vi "RenderTexture.vi"(4 "dstrect":T1, 5 "Entire Rendering Target (F)":bool, 6 "srcrect":T1, 7 "Entire Texture (F)":bool, 8 "No Error":errorcluster, 10 "texture [SDL_Texture *]":i64, 11 "renderer [SDL_Renderer *]":i64) -> (0 "error out":errorcluster)   [LabVIEW 2024, in "SDL3.lvlib" / "Render.lvlib"]
doc: "<B>Summary</B>\nCopy a portion of the texture to the current rendering target at subpixel precision.\n\n<B>Thread Safety</B>\nYou may only call this function from the main thread."
uses:
  Render.lvlib
  Rect/FRect--cluster.ctl
  Error/Error.lvlib
  Lib/SDL3-32.dll
  Rect/Rect.lvlib
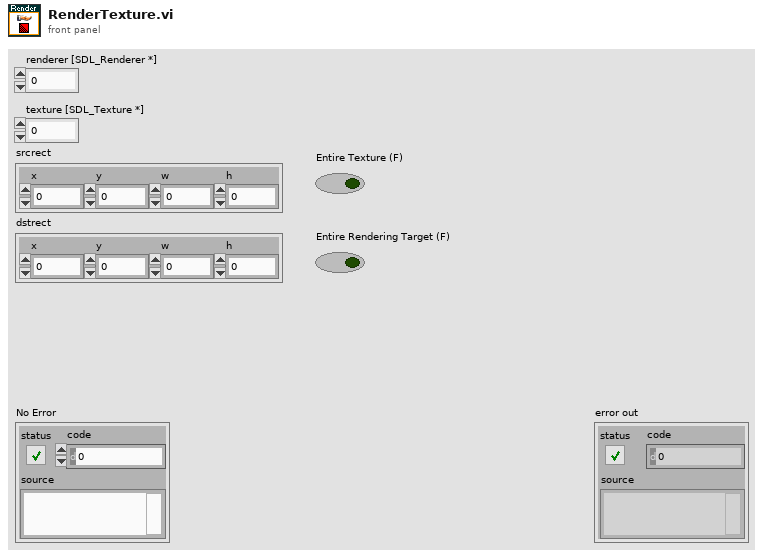
[diagram p1: front panel]
types:
  T1 = typedef "SDL3.lvlib/Rect.lvlib/FRect--cluster.ctl" = cluster{"x":sgl, "y":sgl, "w":sgl, "h":sgl}
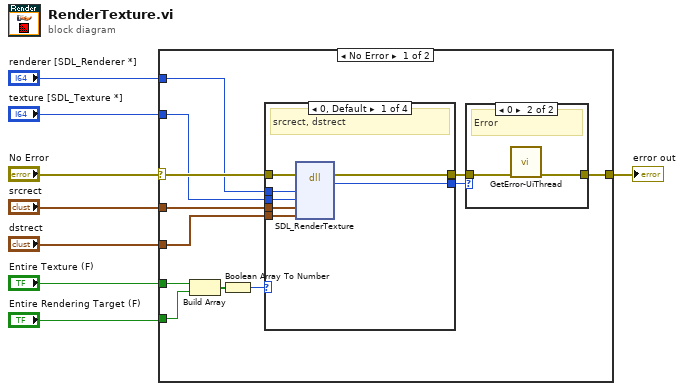
[diagram p0: block diagram]
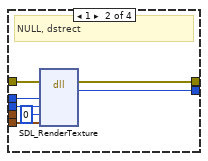
[diagram p2: hidden frame]
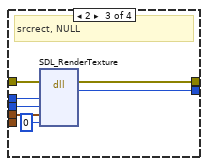
[diagram p3: hidden frame]
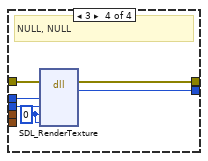
[diagram p4: hidden frame]
diagram:
  n1 = case shown="No Error" "No Error" {
    selector: "No Error" -> [w20 w51]
    tunnel: [w18 w51] -> w7
    tunnel: "renderer [SDL_Renderer *]" -> [w16 _]
    tunnel: "texture [SDL_Texture *]" -> [w15 _]
    tunnel: "srcrect" -> [w14 _]
    tunnel: "dstrect" -> [w13 _]
    tunnel: "Entire Rendering Target (F)" -> [w12 _]
    tunnel: "Entire Texture (F)" -> [w9 _]
    frame No Error {
      n2 = Build Array(w9, w12) -> (w11:bool[])
      n3 = Boolean Array To Number(Boolean array=w11) -> (number=w10:u32)
      n4 = case shown="0, Default" w10 {
        tunnel: w20 -> [w27 w34 w41 w47]
        tunnel: [w26 w33 w40 w46] -> w19
        tunnel: [w25 w32 w39 w45] -> w17
        tunnel: w16 -> [w24 w31 w38 w44]
        tunnel: w15 -> [w23 w30 w37 w43]
        tunnel: w14 -> [w22 _ w36 _]
        tunnel: w13 -> [w21 w28 _ _]
        frame 0, Default {
          # "srcrect, dstrect"
          n5 = dll-call lib="C:/Users/Thomas/Documents/Projects/LV-SDL3/Lib/SDL3-*.*" fn="SDL_RenderTexture"(error in=w27, "renderer"=w24, "texture"=w23, "srcrect"=w22, "dstrect"=w21) -> (error out=w26:errorcluster, "return type"=w25:i32)  [unwired: 6 in, 1 out]
        }
        frame 1 {
          # "NULL, dstrect"
          n6 = dll-call lib="C:/Users/Thomas/Documents/Projects/LV-SDL3/Lib/SDL3-*.*" fn="SDL_RenderTexture"(error in=w34, "renderer"=w31, "texture"=w30, "srcrect"=i64 0 ("dstrect"), "dstrect"=w28) -> (error out=w33:errorcluster, "return type"=w32:i32)  [unwired: 6 in, 1 out]
        }
        frame 2 {
          # "srcrect, NULL"
          n7 = dll-call lib="C:/Users/Thomas/Documents/Projects/LV-SDL3/Lib/SDL3-*.*" fn="SDL_RenderTexture"(error in=w41, "renderer"=w38, "texture"=w37, "srcrect"=w36, "dstrect"=i64 0) -> (error out=w40:errorcluster, "return type"=w39:i32)  [unwired: 6 in, 1 out]
        }
        frame 3 {
          w42 = i64 0 ("dstrect")
          # "NULL, NULL"
          n8 = dll-call lib="C:/Users/Thomas/Documents/Projects/LV-SDL3/Lib/SDL3-*.*" fn="SDL_RenderTexture"(error in=w47, "renderer"=w44, "texture"=w43, "srcrect"=w42, "dstrect"=w42) -> (error out=w46:errorcluster, "return type"=w45:i32)  [unwired: 6 in, 1 out]
        }
      }
      n9 = case shown="0" w17 {
        tunnel: w19 -> [w48 w50]
        tunnel: [w48 w49] -> w18
        frame Default {
          # "Ok"
        }
        frame 0 {
          # "Error"
          n10 = call "GetError-UiThread.vi"("No Error"=w50) -> ("error out"=w49:errorcluster)  [unwired: 10 in]
        }
      }
    }
    frame Error {
    }
  }
  "error out" <- w7
